vi "Electronic Procedure.vi"() -> ()   [LabVIEW 2017]
panel:
  out "Task Tip":string
  out "Experiment Progress":dbl(slide) scale=0.0..44.0
  in  "?":bool
  out "Task 5":bool caption="Vary pump frequency"
  out "Task 4":bool caption="Vary pump frequency"
  out "Task 3":bool caption="Set pump frequency"
  out "Task 1":bool caption="Ensure pump at 0 Hz"
  out "Task 2":bool caption="Phase 2.1 start"
  in  "Array":dbl[](array[numeric])
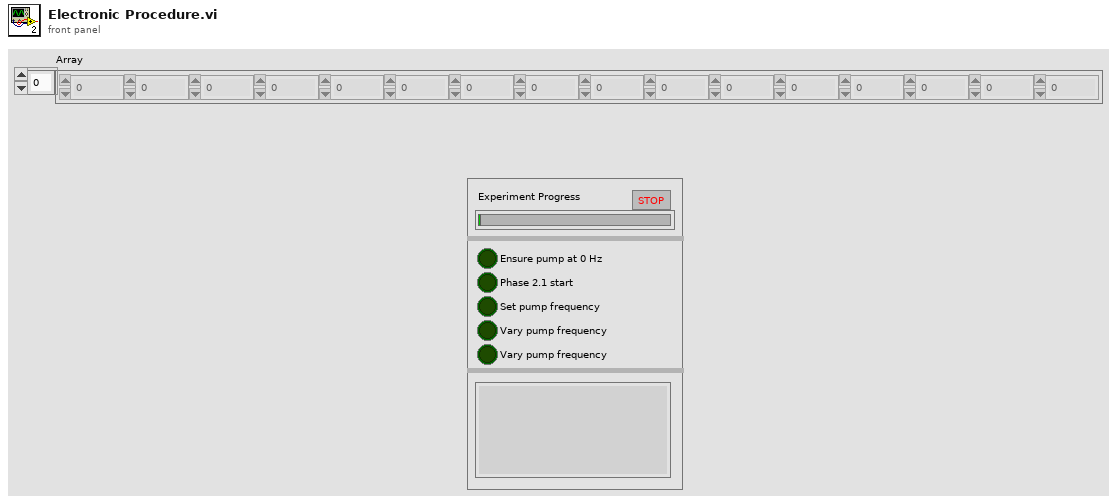
[diagram p1: front panel]
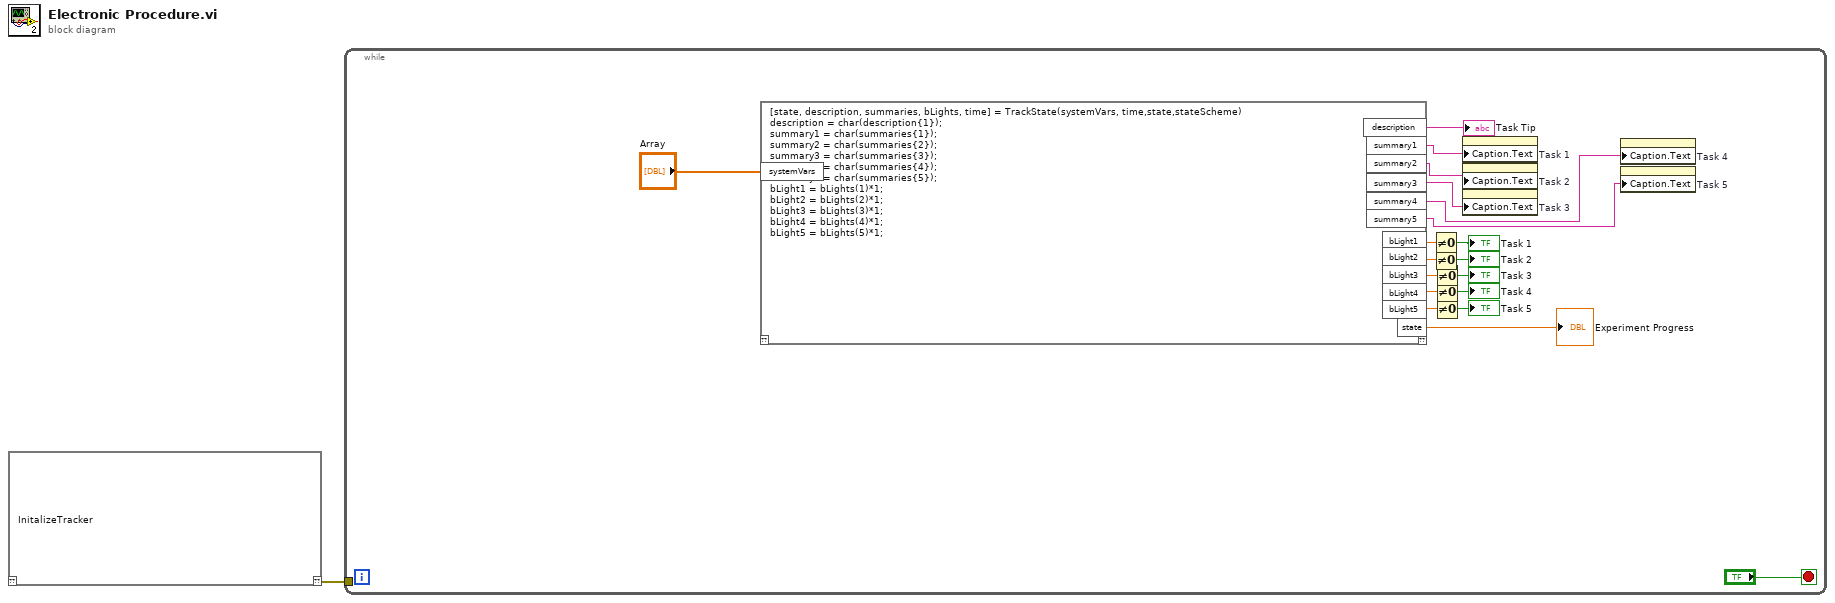
[diagram p0: block diagram]
diagram:
  n1 = script code="InitalizeTracker"() -> ("??"=w1:errorcluster)  [unwired: 1 in]
  n2 = while {
    tunnel: w1 -> [_]
    stop <- "?" stop-if-true
    n3 = script code="[state, description, summaries, bLights, time] = TrackState(systemVars, time,state,stateScheme)\ndescription = char(description{1});\nsummary1 = char(summaries{1});\nsummary2 = char(summaries{2});\nsummary3 = char(summaries{3});\nsummary4 = char(summaries{4});\nsummary5 = char(summaries{5}); \nbLight1 = bLights(1)*1;\nbLight2 = bLights(2)*1;\nbLight3 = bLights(3)*1;\nbLight4 = bLights(4)*1;\nbLight5 = bLights(5)*1;"("systemVars"="Array") -> ("description"=→"Task Tip":string, "summary1"=w6:string, "summary2"=w5:string, "summary3"=w4:string, "summary4"=w3:string, "summary5"=w2:string, "bLight1"=w19:dbl, "bLight2"=w17:dbl, "bLight3"=w14:dbl, "bLight4"=w13:dbl, "bLight5"=w12:dbl, "state"=→"Experiment Progress":dbl)  [unwired: 1 in, 1 out]
    n4 = Not Equal To 0?(x=w19) -> (x != 0?=→"Task 1":bool)
    n5 = Not Equal To 0?(x=w17) -> (x != 0?=→"Task 2":bool)
    n6 = Not Equal To 0?(x=w14) -> (x != 0?=→"Task 3":bool)
    n7 = Not Equal To 0?(x=w13) -> (x != 0?=→"Task 4":bool)
    n8 = Not Equal To 0?(x=w12) -> (x != 0?=→"Task 5":bool)
    n9 = property on="Task 1" class="Bool (strict)"("Caption.Text"=w6) -> ()  [unwired: 2 in, 2 out]
    n10 = property on="Task 2" class="Bool (strict)"("Caption.Text"=w5) -> ()  [unwired: 2 in, 2 out]
    n11 = property on="Task 3" class="Bool (strict)"("Caption.Text"=w4) -> ()  [unwired: 2 in, 2 out]
    n12 = property on="Task 4" class="Bool (strict)"("Caption.Text"=w3) -> ()  [unwired: 2 in, 2 out]
    n13 = property on="Task 5" class="Bool (strict)"("Caption.Text"=w2) -> ()  [unwired: 2 in, 2 out]
  }
